vi "mailError.vi"(1 "Body":string="It works!", 2 "Subject":string="Sending TLS Authenticated Email", 3 "Recipient's Email Address Address":string) -> ()   [LabVIEW 2014]
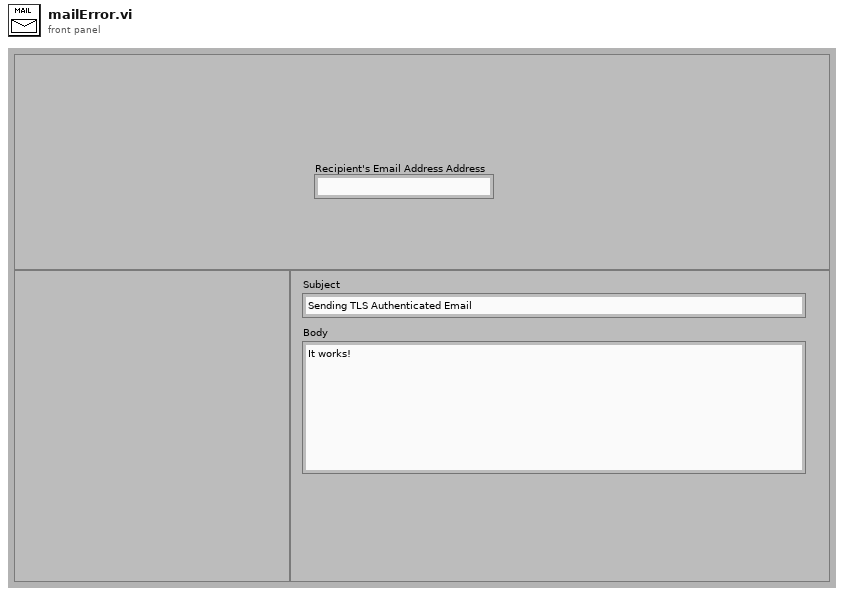
[diagram p1: front panel]
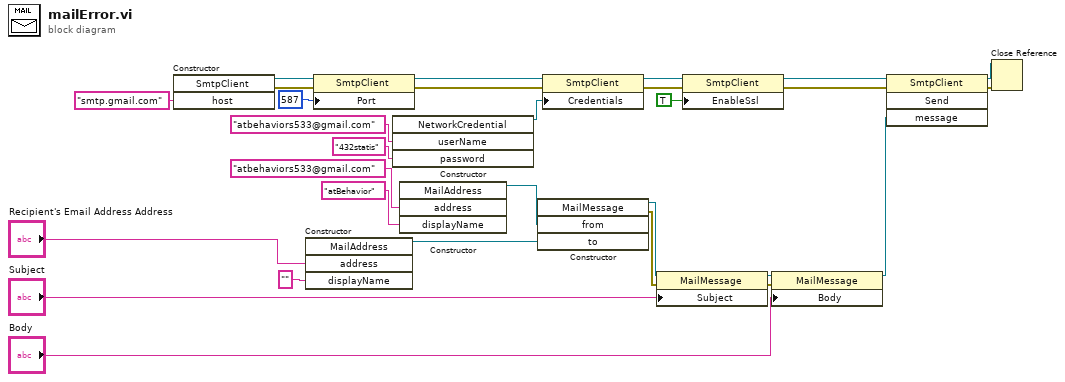
[diagram p0: block diagram]
diagram:
  n1 = constructor class="SmtpClient"("host"="smtp.gmail.com" ("Outgoing Mail Server (SMTP)")) -> (reference out=w14:refnum<k24>, error out=w10:errorcluster)  [unwired: 3 in, 2 out]
  n2 = constructor class="MailAddress"("address"="Recipient's Email Address Address", "displayName"="") -> (reference out=w29:refnum<k24>)  [unwired: 3 in, 4 out]
  n3 = property class="SmtpClient"(reference=w14, error in=w10, "Port"=587) -> (reference out=w13:refnum<k24>, error out=w9:errorcluster)
  n4 = constructor class="NetworkCredential"("userName"="atbehaviors533@gmail.com" ("GMAIL Account User ID (eg: jsmity77)"), "password"="432statis" ("GMAIL Account Password")) -> (reference out=w15:refnum<k24>)  [unwired: 3 in, 4 out]
  n5 = constructor class="MailAddress"("address"="atbehaviors533@gmail.com" ("Sender's Email Address (eg: jsmith77@gmail.com)"), "displayName"="atBehavior" ("Sender's Name")) -> (reference out=w28:refnum<k24>)  [unwired: 3 in, 4 out]
  n6 = constructor class="MailMessage"("from"=w28, "to"=w29) -> (reference out=w3:refnum<k24>, error out=w2:errorcluster)  [unwired: 3 in, 3 out]
  n7 = property class="SmtpClient"(reference=w13, error in=w9, "Credentials"=w15) -> (reference out=w12:refnum<k24>, error out=w8:errorcluster)
  n8 = property class="MailMessage"(reference=w3, error in=w2, "Subject"="Subject") -> (reference out=w20:refnum<k24>, error out=w27:errorcluster)
  n9 = property class="SmtpClient"(reference=w12, error in=w8, "EnableSsl"=TRUE ("Enable SSL")) -> (reference out=w11:refnum<k24>, error out=w7:errorcluster)
  n10 = property class="MailMessage"(reference=w20, error in=w27, "Body"="Body") -> (reference out=w4:refnum<k24>)  [unwired: 1 out]
  n11 = invoke class="SmtpClient" method="Send"(reference=w11, error in=w7, "message"=w4) -> (reference out=w6:refnum<k24>, error out=w5:errorcluster)  [unwired: 1 in, 2 out]
  n12 = Close Reference(reference=w6, error in (no error)=w5) -> ()  [unwired: 1 out]
